vi "Read Events Registrants.vi"(8 "Error In":errorcluster, 11 "Event Source In":refnum<class "Event Source.lvclass">) -> (0 "Error Out":errorcluster, 2 "Events Registrants":T1(c390), 3 "Event Source Out":refnum<class "Event Source.lvclass">)   [LabVIEW 2019, in "Event Source.lvlib" / "Event Source.lvclass"]
doc: "This method returns a map of all subscriptions and can be used to understand more about which actors are subscribed for which events."
uses:
  Event Source.lvclass
  Event Source Messages/Event Generated Msg/Event Generated Msg.lvclass
  <vilib>/ActorFramework/Message Enqueuer/Message Enqueuer.lvclass
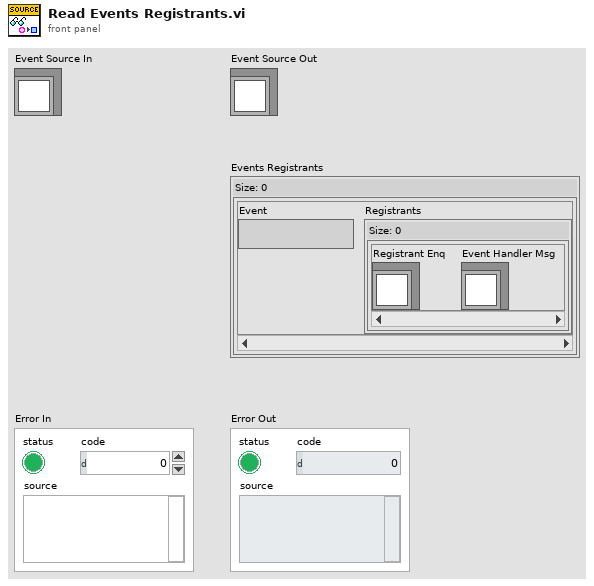
[diagram p1: front panel]
types:
  T1 = map{string, map{refnum<class "Message Enqueuer.lvclass">, refnum<class "Event Generated Msg.lvclass">}}
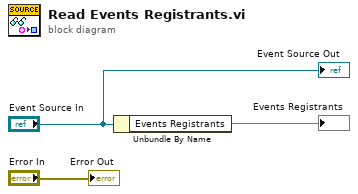
[diagram p0: block diagram]
diagram:
  n1 = Unbundle By Name("Event Source In") -> ("Events Registrants"=→"Events Registrants":T1)
  "Event Source Out" <- "Event Source In"
  "Error Out" <- "Error In"
